vi "OAT Order Magnitude and Phase (Even Angle Signal, N Channels).vi"(0 "even-angle signals":cluster{"r0":dbl, "dr":dbl, "Y":dbl[]}[](array[cluster]) {"r0" format="%.2p"; "dr" format="%.2p"; "Y" format="%.2f"}, 1 "x-axis selection":u16(ring)=2 items=["Time", "Revolution", "RPM"], 2 "reset? (F)":bool, 5 "even-angle channel info":T9[](array[typedef]) {"channel info"."pregain" format="%.2f"; "channel info"."weighting filter" items=["Linear", "A-weighting", "B-weighting", "C-weighting", "ITU-R 468-4", "Dolby", "CCITT", "C-message", "Wb", "Wc", "Wd", "We", "Wf", "Wh", "Wj", "Wk", "Wm", "AES17 20 kHz lowpass", "AES17 40 kHz lowpass", "AES17 20 kHz highpass", "AES17 40 kHz highpass"]; "channel info"."dB reference" format="%^.1e"; "channel info"."engineering units" items=["custom..."=0, "V"=1, "A"=21, "C"=30, "pC"=31, "s"=32, "-"=29, "Pa"=2, "N"=20, "g"=3, "m/s^2"=4, "m/s"=5, "m"=6, "mm/s"=12, "mm"=13, "micron/s"=14, "micron"=15, "in/s^2"=7, "in/s"=8, "in"=9, "mil/s"=10, "mil"=11, "rad/s^2"=16, "rad/s"=17, "rad"=18, "deg/s^2"=26, "deg/s"=27, "deg"=28, "RPM"=22, "cycle/s^2"=23, "Hz"=24, "cycle"=25, "strain"=19]; "channel info"."sensor sensitivity" format="%#_5f"}, 7 "even-angle position info":T1, 9 "orders to compute (1.0)":dbl[](array[numeric])=[1.0] format="%.2f", 11 "error in (no error)":errorcluster, 12 "bandwidth [order]":dbl=1.0 format="%.2f", 13 "view":T12={"dB on? (F)"=FALSE, "unwrap phase? (T)"=TRUE, "unit in degree? (T)"=TRUE}, 14 "zero delay? (F)":bool) -> (3 "unit labels":T8(array[cluster]), 4 "magnitudes [RMS]":T11(array[cluster]) {"magnitude" format="%.2f"; "time/rev/rpm" format="%.2f"}, 6 "phases [phase lag]":cluster{"time/rev/rpm":dbl[], "phase":dbl[]}[][](array[cluster]) {"phase" format="%.2f"; "time/rev/rpm" format="%.2f"}, 8 "magnitude/phase position info":T1, 10 "magnitudes info":T2[](array[typedef]) {"x-axis units" items=["Time (s)"=0, "Frequency-CB (Hz)"=1, "Frequency-CPB (Hz)"=1248, "Frequency-Arbitrary (Hz)"=2357, "Quefrency (s)"=2, "Revolutions (rev)"=3, "Order"=4, "Speed (RPM)"=11, "Speed (rad/s)"=21, "Index"=65535]; "weighting filter" items=["Linear", "A-weighting", "B-weighting", "C-weighting", "ITU-R 468-4", "Dolby", "CCITT", "C-message", "Wb", "Wc", "Wd", "We", "Wf", "Wh", "Wj", "Wk", "Wm", "AES17 20 kHz lowpass", "AES17 40 kHz lowpass", "AES17 20 kHz highpass", "AES17 40 kHz highpass"]; "dB reference [EU]" format="%.2f"; "engineering units" items=["custom..."=0, "V"=1, "A"=21, "C"=30, "pC"=31, "s"=32, "-"=29, "Pa"=2, "N"=20, "g"=3, "m/s^2"=4, "m/s"=5, "m"=6, "mm/s"=12, "mm"=13, "micron/s"=14, "micron"=15, "in/s^2"=7, "in/s"=8, "in"=9, "mil/s"=10, "mil"=11, "rad/s^2"=16, "rad/s"=17, "rad"=18, "deg/s^2"=26, "deg/s"=27, "deg"=28, "RPM"=22, "cycle/s^2"=23, "Hz"=24, "cycle"=25, "strain"=19]; "spectral info"."window" items=["None "=0, "Hanning"=1, "Hamming"=2, "Blackman-Harris"=3, "Exact Blackman"=4, "Blackman"=5, "Flat Top"=6, "4 Term B-Harris "=7, "7 Term B-Harris"=8, "Low Sidelobe"=9, "Force - Exponential"=10, "Gaussian"=62]}, 15 "error out":errorcluster)   [LabVIEW 2017, in "SoundVib_OrderTracking.lvlib"]
doc: "Computes the magnitudes and phases of designated orders in an even-angle signal. Use this VI to track particular orders specified by <B>orders to compute</B>. Wire data to the <B>even-angle signal</B> input to determine the polymorphic instance to use or manually select the instance."
uses:
  <vilib>/addons/Sound and Vibration/Order Analysis/Resample Order Tracking/SoundVib_OrderTracking.lvlib
  <vilib>/addons/Sound and Vibration/Order Analysis/Misc/OAT Position Info.ctl
  <vilib>/addons/_NISVFA/_Shared subVIs/Controls/svc_Resampled Channel Info.ctl
  <vilib>/addons/_NISVFA/_Shared subVIs/Controls/svc_Channel Info.ctl
  <vilib>/addons/_NISVFA/_Shared subVIs/Controls/svc_Engineering Units Text Ring.ctl
  <vilib>/addons/_NISVFA/_Shared subVIs/Controls/svc_Weighting Filter Text Ring.ctl
  <vilib>/addons/_NISVFA/_Shared subVIs/Controls/svc_Spectrum Info.ctl
  <vilib>/addons/_NISVFA/_Shared subVIs/Controls/svc_X-Axis Units.ctl
  <vilib>/addons/_NISVFA/_Shared subVIs/Controls/svc_Spectrum Type.ctl
  <vilib>/addons/_NISVFA/_Shared subVIs/Controls/svc_Complimentary Spectrum Units.ctl
  <vilib>/addons/Sound and Vibration/Order Analysis/Resample Order Tracking/SubVIs/OAT Order Magnitude and Phase Plot(XY) (Multi Channels).vi
  <vilib>/addons/Sound and Vibration/Order Analysis/Resample Order Tracking/SubVIs/OAT Demodulate Multiple Orders (Multi Channels).vi
  <vilib>/addons/Sound and Vibration/Order Analysis/Resample Order Tracking/SubVIs/OAT Verify Resampled Signal (OMP, Multi Channels).vi
  <vilib>/addons/Sound and Vibration/Order Analysis/Resample Order Tracking/SoundVib_Resampling.lvlib
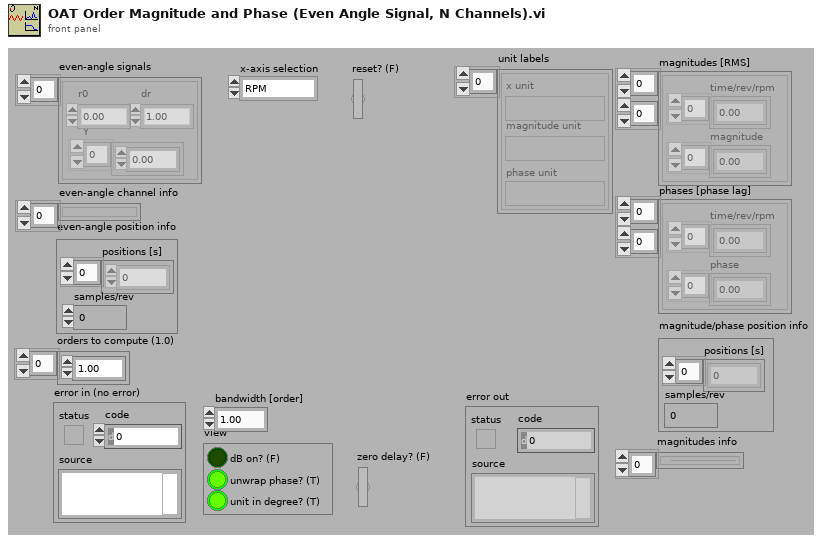
[diagram p1: front panel]
types:
  T1 = typedef "OAT Position Info.ctl" = cluster{"positions [s]":dbl[], "samples/rev":dbl}
  T2 = typedef "svc_Spectrum Info.ctl" = cluster{"channel name":string, "description":string, "x-axis units":T3, "spectral info":cluster{"spectrum type":T4, "linear/dB":enum16{"linear", "dB"}, "window":u16, "window size":i32, "FFT size":i32}, "engineering units":T5, "custom label":string, "dB reference [EU]":dbl, "peak units":enum16{"rms", "peak", "peak-peak"}, "weighting filter":T6, "spectral density?":bool, "unit label":string, "spectrum skewed?":bool, "complimentary spectrum units":T7}
  T3 = typedef "svc_X-Axis Units.ctl" = u16
  T4 = typedef "svc_Spectrum Type.ctl" = enum16{"FFT Spectrum [complex]", "Amplitude [Magnitude]", "Power [Magnitude^2]", "Cross Spectrum [complex]", "Frequency Response [Complex]"}
  T5 = typedef "svc_Engineering Units Text Ring.ctl" = u16
  T6 = typedef "svc_Weighting Filter Text Ring.ctl" = u16
  T7 = typedef "svc_Complimentary Spectrum Units.ctl" = enum16{"none", "radians", "degrees", "cycles", "imaginary"}
  T8 = cluster{"x unit":string, "magnitude unit":string, "phase unit":string}[]
  T9 = typedef "svc_Resampled Channel Info.ctl" = cluster{"channel name":string, "description":string, " channel info":T10}
  T10 = typedef "svc_Channel Info.ctl" = cluster{"sensor sensitivity":dbl, "engineering units":T5, "dB reference":dbl, "custom label":string, "weighting filter":T6, "pregain":dbl}
  T11 = cluster{"time/rev/rpm":dbl[], "magnitude":dbl[]}[][]
  T12 = cluster{"dB on? (F)":bool, "unwrap phase? (T)":bool, "unit in degree? (T)":bool}
  T13 = cluster{"X unit":string, "unit label":string, "unit label":string}[]
  T14 = cluster{"bandwidth [order] out":dbl, "stop band attenuation":u16}
  T15 = cluster{"unwrap phase? (T)":bool, "unit in degree? (T)":bool}
  T16 = typedef "SoundVib_TachProcess.lvlib/speed profile.ctl" = cluster{"time [s]":dbl[], "speed [RPM]":dbl[]}
  T17 = cluster{"X unit":string, "unit label":string, "unit label":string}
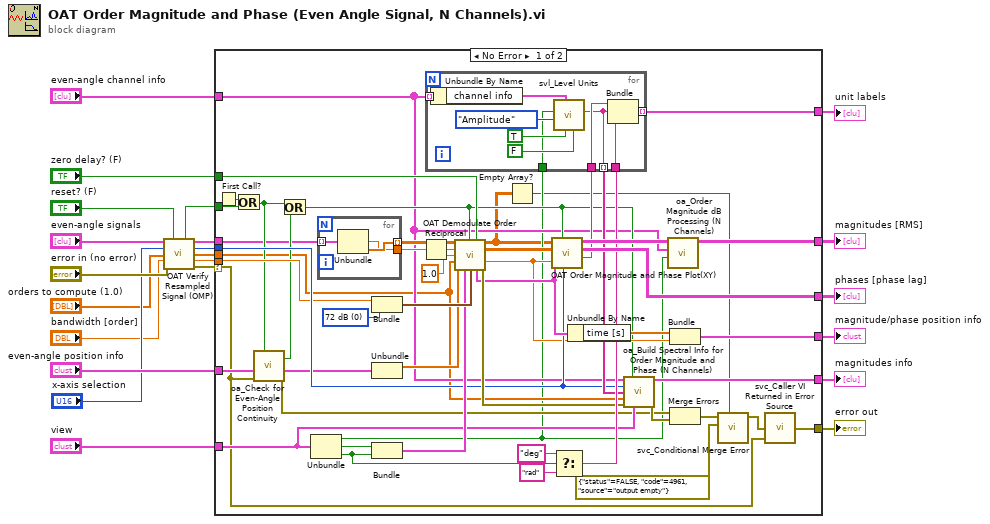
[diagram p0: block diagram]
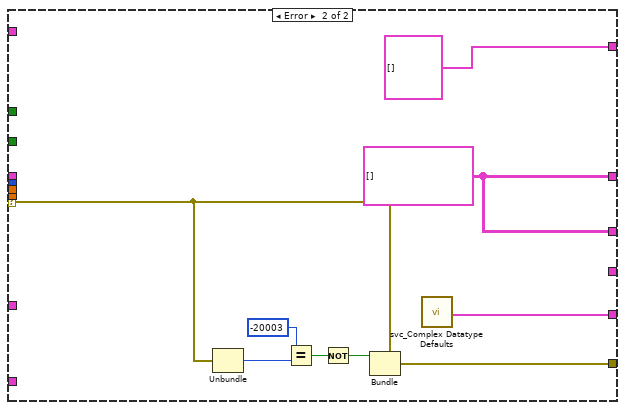
[diagram p2: hidden frame]
diagram:
  n1 = call-poly <vilib>:"OAT Verify Resampled Signal (OMP).vi"("resampled signal"="even-angle signals", "reset in (T)"="reset? (F)", "X axis selection"="x-axis selection", "orders to compute (1.0)"="orders to compute (1.0)", "bandwidth [order]"="bandwidth [order]", "error in (no error)"="error in (no error)") -> ("reset out (T)"=w9:bool, "resampled signal out"=w12:cluster{"r0":dbl, "dr":dbl, "Y":dbl[]}[], "X axis selection out"=w7:u16, "orders to compute (1.0) out"=w3:dbl[], "bandwidth [order] out"=w5:dbl, "error out"=w11:errorcluster)  [unwired: 4 in]
  n2 = case shown="No Error" w11 {
    selector: w11 -> [w23 w90]
    tunnel: [w70 T13 []] -> w16
    tunnel: "even-angle position info" -> [w33 _]
    tunnel: "view" -> [w43 _]
    tunnel: [w72 w94] -> w20
    tunnel: [w49 w94] -> w19
    tunnel: w9 -> [w47 _]
    tunnel: [w24 w87] -> w18
    tunnel: "even-angle channel info" -> [w35 _]
    tunnel: [w69 w86] -> w15
    tunnel: [w68 _] -> w14
    tunnel: w12 -> [w34 _]
    tunnel: w7 -> [w46 _]
    tunnel: w5 -> [w45 _]
    tunnel: w3 -> [w31 _]
    tunnel: "zero delay? (F)" -> [w40 _]
    frame No Error {
      w55 = u16 0 items=["72 dB", "96 dB", "120 dB"] ("stop band attenuation")
      n3 = First Call?() -> (First Call?: T/F=w48:bool)
      n4 = Or(x=w48, y=w47) -> (x .or. y?=w39:bool)
      n5 = call <vilib>:"oa_Check for Even-Angle Position Continuity.vi"("reset in"=w39, "error in (no error)"=w23, "even-angle position info"=w33) -> ("error out"=w36:errorcluster, "even-angle position info dup"=w32:T1, "position not continuous"=w38:bool)  [unwired: 6 in]
      n6 = Or(x=w39, y=w38) -> (x .or. y?=w37:bool)
      n7 = Unbundle(w43) -> ("dB on? (F)"=w30:bool, "unwrap phase? (T)"=w51:bool, "unit in degree? (T)"=w44:bool)
      n8 = for {
        tunnel: w34 -> [w75] mode=indexing
        tunnel: [w74] -> w60 mode=indexing
        tunnel: [w73] -> w61
        n9 = Unbundle(w75) -> ("dr"=w73:dbl, "Y"=w74:dbl[])  [unwired: 1 out]
      }
      n10 = Bundle("bandwidth [order] out"=w45, "stop band attenuation"=w55) -> (w56:T14)  [unwired: 1 in]
      n11 = Unbundle(w32) -> ("positions [s]"=w53:dbl[])  [unwired: 1 out]
      n12 = Bundle("unwrap phase? (T)"=w51, "unit in degree? (T)"=w44) -> (w50:T15)  [unwired: 1 in]
      n13 = Reciprocal(x=w61) -> (1/x=w59:dbl)
      n14 = call-poly <vilib>:"OAT Demodulate Order.vi"("Y"=w60, "reset? (True)"=w37, "zero delay? (F)"=w40, "samples/rev"=w59, "samples/rev wanted"=1.0 ("x"), "orders (1.0)"=w31, "time stamps in"=w53, "phase setting"=w50, "order info"=w56) -> ("magnitudes (RMS)"=w27:dbl[][][], "phase lag"=w63:dbl[][][], "samples/rev"=w42:dbl, "speed profile"=w54:T16, "error out"=w58:errorcluster)  [unwired: 2 in]
      n15 = Empty Array?(array=w27) -> (empty?=w26:bool)
      n16 = call-poly <vilib>:"OAT Order Magnitude and Phase Plot(XY).vi"("X axis selection"=w46, "reset? (True)"=w37, "speed profile"=w54, "samples/rev"=w42, "phase lag  (even angular)"=w63, "magnitudes (even angular)"=w27) -> ("X unit"=w65:string, "phase lag"=w72:cluster{"X":dbl[], "Y":dbl[]}[][], "magnitudes"=w71:cluster{"X":dbl[], "Y":dbl[]}[][])  [unwired: 3 in]
      n17 = Select(t="deg" ("unit label"), s=w44, f="rad" ("unit label")) -> (s? t:f=w64:string)
      n18 = for {
        tunnel: w65 -> [w85]
        tunnel: w64 -> [w84]
        tunnel: [w83] -> w70 mode=indexing
        tunnel: w35 -> [w81] mode=indexing
        tunnel: [w79] -> w57 mode=indexing
        tunnel: w30 -> [w76]
        n19 = Unbundle By Name(w81) -> ("channel info"=w80:T10)
        n20 = call <vilib>:"svl_Level Units.vi"("include weighting if dB On FALSE"=FALSE, "rms level (T)"=TRUE, "channel info"=w80, "view mode"=enum16{"Power", "Amplitude"}."Amplitude", "dB On (T)"=w76) -> ("unit label"=w79:string)  [unwired: 4 in, 2 out]
        n21 = Bundle("X unit"=w85, "unit label"=w79, "unit label"=w84) -> (w83:T17)  [unwired: 1 in]
      }
      n22 = Unbundle By Name(w54) -> ("time [s]"=w52:dbl[])
      n23 = call <vilib>:"oa_Build Spectral Info for Order Magnitude and Phase (N Channels).vi"("channel info"=w35, "reset? (T)"=w37, "X axis selection"=w46, "unit labels"=w57, "orders to compute"=w31, "error in (no error)"=w58, "view"=w43) -> ("spectrum info"=w69:T2[], "error out"=w41:errorcluster)  [unwired: 7 in]
      n24 = call <vilib>:"oa_Order Magnitude dB Processing (N Channels).vi"("dB on? (T)"=w30, "even angle channel info"=w35, "magnitudes"=w71) -> ("magnitudes dB"=w49:cluster{"X":dbl[], "Y":dbl[]}[][])  [unwired: 8 in]
      n25 = Bundle("time [s]"=w52, "samples/rev"=w42) -> (w68:cluster{"time [s]":dbl[], "samples/rev":dbl})  [unwired: 1 in]
      n26 = Merge Errors(w36, w41) -> (w28:errorcluster)
      n27 = call <vilib>:"svc_Conditional Merge Error.vi"("merge"=w26, "new error"=errorcluster {"status"=FALSE, "code"=4961, "source"="output empty"}, "error in (no error)"=w28) -> ("error out"=w25:errorcluster)  [unwired: 8 in]
      n28 = call <vilib>:"svc_Caller VI Returned in Error Source.vi"("warning input to caller"=w23, "error in (no error)"=w25) -> ("error out"=w24:errorcluster)  [unwired: 3 in]
    }
    frame Error {
      w94 = cluster{"X":dbl[], "Y":dbl[]}[][] [] ("magnitudes")
      n29 = Unbundle(w90) -> ("code"=w92:i32)  [unwired: 2 out]
      n30 = Equal?(x=-20003 ("t"), y=w92) -> (x = y?=w89:bool)
      n31 = Not(x=w89) -> (.not. x?=w88:bool)
      n32 = Bundle(cluster=w90, "status"=w88) -> (w87:errorcluster)  [unwired: 2 in]
      n33 = call <vilib>:"svc_Complex Datatype Defaults.vi"() -> ("empty array of spectrum info"=w86:T2[])  [unwired: 11 in, 8 out]
    }
  }
  "magnitudes [RMS]" <- w19
  "phases [phase lag]" <- w20
  "error out" <- w18
  "unit labels" <- w16
  "magnitudes info" <- w15
  "magnitude/phase position info" <- w14
